vi "getStatusEotFwd.vi"(8 "error in":errorcluster, 9 "Status EOT FWD in":bool=TRUE, 10 "axis in":u8, 11 "connection ID":refnum<k5>) -> (0 "error out":errorcluster, 1 "Status EOT FWD out":bool=TRUE, 2 "axis out":u8, 3 "connection ID":refnum<k5>)   [LabVIEW 2019]
panel:
  in  "Get Command":string="com.attocube.amc.status.getStatusEotFwd"
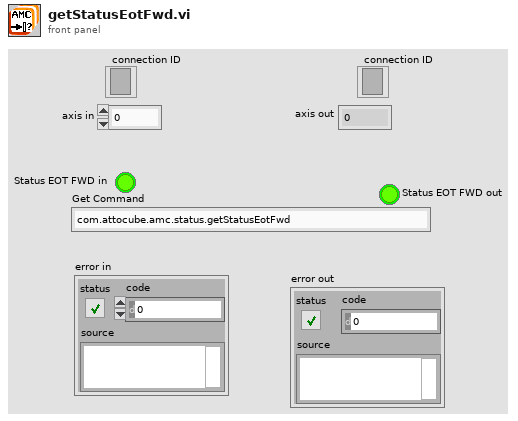
[diagram p1: front panel]
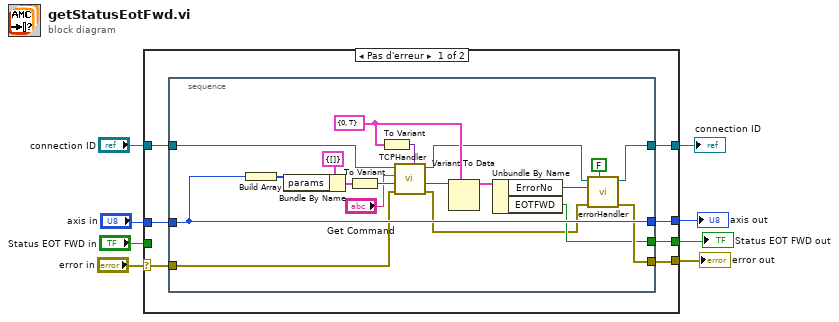
[diagram p0: block diagram]
diagram:
  n1 = case shown="Pas d'erreur" "error in" {
    selector: "error in" -> [w9 w36]
    tunnel: "axis in" -> [w11 w38]
    tunnel: [w15 w36] -> w7
    tunnel: [w14 w38] -> w6
    tunnel: [w12 w37] -> w5
    tunnel: [w13 w35] -> w4
    tunnel: "connection ID" -> [w10 w35]
    tunnel: "Status EOT FWD in" -> [_ w37]
    frame No Error {
      n2 = stacked-sequence {
        tunnel: [w19] -> w13
        tunnel: w10 -> [w24]
        tunnel: w11 -> [w26]
        tunnel: [w26] -> w14
        tunnel: [w21] -> w12
        tunnel: [w25] -> w15
        tunnel: w9 -> [w17]
        frame #0 {
          w22 = cluster{"ErrorNo":i32, "EOTFWD":bool} {"ErrorNo"=0, "EOTFWD"=TRUE} ("input cluster")
          n3 = Build Array(w26) -> (w30:u8[])
          n4 = Bundle By Name(cluster=cluster{"params":i32[]} {"params"=[]} ("input cluster"), "params"=w30) -> (w31:cluster{"params":i32[]})
          n5 = To Variant(anything=w31) -> (Variant=w32:variant)
          n6 = To Variant(anything=w22) -> (Variant=w23:variant)
          n7 = call <userlib>:"TCPHandler.vi"("result Types"=w23, "error in (no error)"=w17, "params"=w32, "method"="Get Command", "connection ID"=w24) -> ("error out"=w16:errorcluster, "result"=w28:variant, "connection ID"=w20:refnum<k5>)  [unwired: 3 in, 1 out]
          n8 = Variant To Data(type=w22, Variant=w28) -> (data=w33:cluster{"ErrorNo":i32, "EOTFWD":bool})  [unwired: 1 in, 1 out]
          n9 = Unbundle By Name(w33) -> ("ErrorNo"=w34:i32, "EOTFWD"=w21:bool)
          n10 = call <userlib>:"errorHandler.vi"("show popup"=FALSE, "error in"=w16, "error number"=w34, "connection ID"=w20) -> ("error out"=w25:errorcluster, "connection ID"=w19:refnum<k5>)  [unwired: 6 in]
        }
      }
    }
    frame Error {
    }
  }
  "error out" <- w7
  "axis out" <- w6
  "Status EOT FWD out" <- w5
  "connection ID" <- w4
